vi "LEDSA --DOWN--.vi"(2 "Error In":errorcluster, 3 "FPGA VI Reference In":refnum<k20>) -> (0 "Error Out":errorcluster, 1 "FPGA VI Reference Out":refnum<k20>)   [LabVIEW 2015]
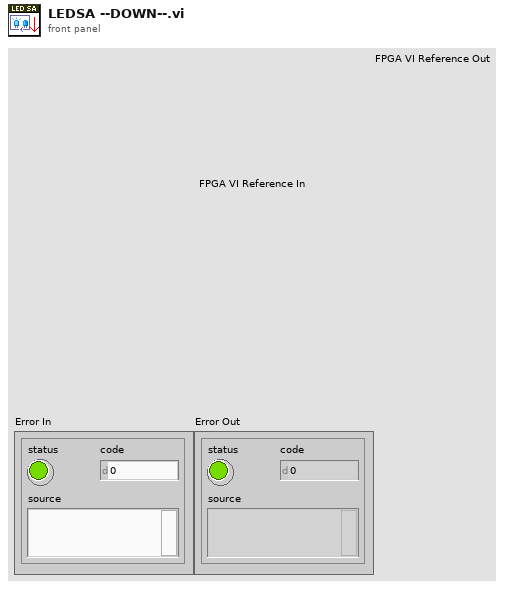
[diagram p1: front panel]
types:
  T1 = cluster{"LED 3":enum16{"Brightness", "Bool"}, "BOOL":bool, "Brightness":u32}
  T2 = cluster{"LED 1":enum16{"Brightness", "Bool"}, "BOOL":bool, "Brightness":u32}
  T3 = cluster{"LED 2":enum16{"Brightness", "Bool"}, "BOOL":bool, "Brightness":u32}
  T4 = cluster{"LED 0":enum16{"Brightness", "Bool"}, "BOOL":bool, "Brightness":u32}
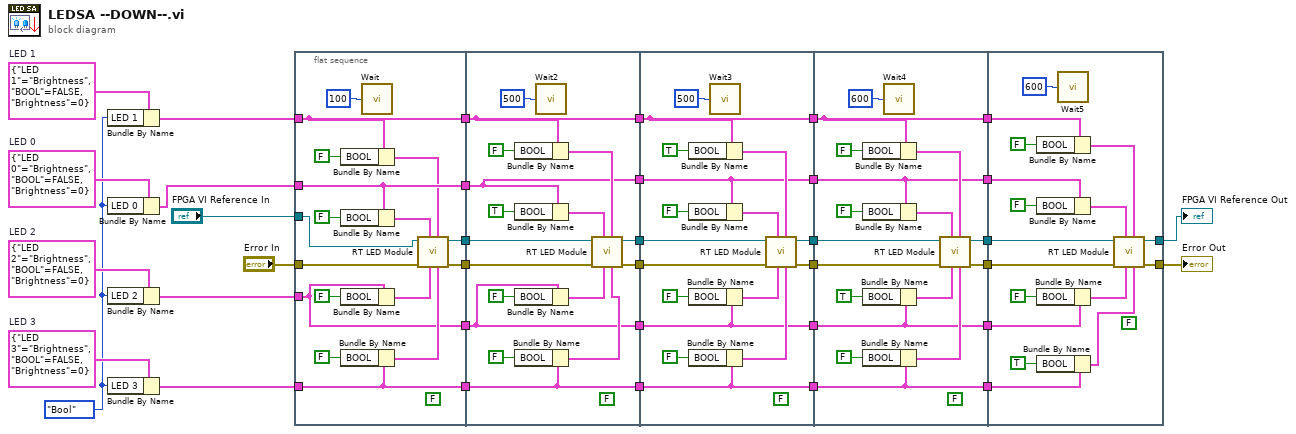
[diagram p0: block diagram]
diagram:
  w18 = T1 {"LED 3"=enum."Brightness", "BOOL"=FALSE, "Brightness"=0}  # LED 3
  w21 = T2 {"LED 1"=enum."Brightness", "BOOL"=FALSE, "Brightness"=0}  # LED 1
  w19 = T3 {"LED 2"=enum."Brightness", "BOOL"=FALSE, "Brightness"=0}  # LED 2
  w20 = T4 {"LED 0"=enum."Brightness", "BOOL"=FALSE, "Brightness"=0}  # LED 0
  w17 = enum16{"Brightness", "Bool"}."Bool" ("LED")
  n1 = Bundle By Name(cluster=w21, "LED 1"=w17) -> (w15:T2)
  n2 = Bundle By Name(cluster=w20, "LED 0"=w17) -> (w16:T4)
  n3 = Bundle By Name(cluster=w19, "LED 2"=w17) -> (w14:T3)
  n4 = Bundle By Name(cluster=w18, "LED 3"=w17) -> (w13:T1)
  n5 = flat-sequence {
    tunnel: [w54] -> w37
    tunnel: "Error In" -> [w52]
    tunnel: [w48] -> w36
    tunnel: [w46] -> w35
    tunnel: [w45] -> w34
    tunnel: [w44] -> w33
    tunnel: w16 -> [w48]
    tunnel: w15 -> [w46]
    tunnel: w14 -> [w45]
    tunnel: w13 -> [w44]
    tunnel: [w39] -> w2
    tunnel: "FPGA VI Reference In" -> [w38]
    tunnel: w37 -> [w70]
    tunnel: [w71] -> w32
    tunnel: w36 -> [w64]
    tunnel: [w64] -> w31
    tunnel: w35 -> [w63]
    tunnel: [w63] -> w30
    tunnel: w34 -> [w62]
    tunnel: [w62] -> w29
    tunnel: w33 -> [w61]
    tunnel: [w61] -> w28
    tunnel: [w56] -> w3
    tunnel: w2 -> [w55]
    tunnel: w32 -> [w87]
    tunnel: [w88] -> w27
    tunnel: w31 -> [w81]
    tunnel: [w81] -> w26
    tunnel: w30 -> [w80]
    tunnel: [w80] -> w25
    tunnel: w29 -> [w79]
    tunnel: [w79] -> w24
    tunnel: w28 -> [w78]
    tunnel: [w78] -> w23
    tunnel: [w73] -> w4
    tunnel: w3 -> [w72]
    tunnel: w27 -> [w104]
    tunnel: w26 -> [w93]
    tunnel: w25 -> [w94]
    tunnel: w24 -> [w92]
    tunnel: w23 -> [w91]
    tunnel: [w105] -> w12
    tunnel: [w94] -> w11
    tunnel: [w93] -> w10
    tunnel: [w92] -> w9
    tunnel: [w91] -> w8
    tunnel: [w90] -> w5
    tunnel: w4 -> [w89]
    tunnel: w12 -> [w107]
    tunnel: w11 -> [w110]
    tunnel: w10 -> [w111]
    tunnel: w9 -> [w112]
    tunnel: w8 -> [w113]
    tunnel: [w109] -> w7
    tunnel: [w108] -> w6
    tunnel: w5 -> [w106]
    frame #0 {
      (unwired) FALSE ("Stop Button")
      n6 = Bundle By Name(cluster=w46, "BOOL"=FALSE) -> (w47:T2)
      n7 = Bundle By Name(cluster=w48, "BOOL"=FALSE) -> (w51:T4)
      n8 = Bundle By Name(cluster=w45, "BOOL"=FALSE) -> (w50:T3)
      n9 = Bundle By Name(cluster=w44, "BOOL"=FALSE) -> (w49:T1)
      n10 = call "Wait"("Count(mSec)"=u32 100) -> ()  [unwired: 1 out]
      n11 = call "RT LED Module.vi"("LED 3"=w49, "LED 1"=w47, "LED 2"=w50, "LED 0"=w51, "error in"=w52, "FPGA VI Reference In"=w38) -> ("error out"=w54:errorcluster, "FPGA VI Reference Out"=w39:refnum<k20>)  [unwired: 4 in]
    }
    frame #1 {
      (unwired) FALSE ("Stop Button")
      n12 = Bundle By Name(cluster=w63, "BOOL"=FALSE) -> (w68:T2)
      n13 = Bundle By Name(cluster=w64, "BOOL"=TRUE) -> (w67:T4)
      n14 = Bundle By Name(cluster=w62, "BOOL"=FALSE) -> (w65:T3)
      n15 = Bundle By Name(cluster=w61, "BOOL"=FALSE) -> (w66:T1)
      n16 = call "Wait2"("Count(mSec)"=u32 500) -> ()  [unwired: 1 out]
      n17 = call "RT LED Module.vi"("LED 3"=w66, "LED 1"=w68, "LED 2"=w65, "LED 0"=w67, "error in"=w70, "FPGA VI Reference In"=w55) -> ("error out"=w71:errorcluster, "FPGA VI Reference Out"=w56:refnum<k20>)  [unwired: 4 in]
    }
    frame #2 {
      (unwired) FALSE ("Stop Button")
      n18 = Bundle By Name(cluster=w80, "BOOL"=TRUE) -> (w83:T2)
      n19 = Bundle By Name(cluster=w81, "BOOL"=FALSE) -> (w82:T4)
      n20 = Bundle By Name(cluster=w79, "BOOL"=FALSE) -> (w84:T3)
      n21 = Bundle By Name(cluster=w78, "BOOL"=FALSE) -> (w85:T1)
      n22 = call "Wait3"("Count(mSec)"=u32 500) -> ()  [unwired: 1 out]
      n23 = call "RT LED Module.vi"("LED 3"=w85, "LED 1"=w83, "LED 2"=w84, "LED 0"=w82, "error in"=w87, "FPGA VI Reference In"=w72) -> ("error out"=w88:errorcluster, "FPGA VI Reference Out"=w73:refnum<k20>)  [unwired: 4 in]
    }
    frame #3 {
      (unwired) FALSE ("Stop Button")
      n24 = Bundle By Name(cluster=w94, "BOOL"=FALSE) -> (w101:T2)
      n25 = Bundle By Name(cluster=w93, "BOOL"=FALSE) -> (w102:T4)
      n26 = Bundle By Name(cluster=w92, "BOOL"=TRUE) -> (w100:T3)
      n27 = Bundle By Name(cluster=w91, "BOOL"=FALSE) -> (w99:T1)
      n28 = call "Wait4"("Count(mSec)"=u32 600) -> ()  [unwired: 1 out]
      n29 = call "RT LED Module.vi"("LED 3"=w99, "LED 1"=w101, "LED 2"=w100, "LED 0"=w102, "error in"=w104, "FPGA VI Reference In"=w89) -> ("error out"=w105:errorcluster, "FPGA VI Reference Out"=w90:refnum<k20>)  [unwired: 4 in]
    }
    frame #4 {
      (unwired) FALSE ("Stop Button")
      n30 = Bundle By Name(cluster=w110, "BOOL"=FALSE) -> (w116:T2)
      n31 = Bundle By Name(cluster=w111, "BOOL"=FALSE) -> (w115:T4)
      n32 = Bundle By Name(cluster=w112, "BOOL"=FALSE) -> (w117:T3)
      n33 = Bundle By Name(cluster=w113, "BOOL"=TRUE) -> (w118:T1)
      n34 = call "Wait5"("Count(mSec)"=u32 600) -> ()  [unwired: 1 out]
      n35 = call "RT LED Module.vi"("LED 3"=w118, "LED 1"=w116, "LED 2"=w117, "LED 0"=w115, "error in"=w107, "FPGA VI Reference In"=w106) -> ("error out"=w109:errorcluster, "FPGA VI Reference Out"=w108:refnum<k20>)  [unwired: 4 in]
    }
  }
  "Error Out" <- w7
  "FPGA VI Reference Out" <- w6
